vi "orientation_tester.vi"() -> ()   [LabVIEW 2026]
uses:
  <vilib>/Utility/error.llb/Trim Whitespace One-Sided.vi
panel:
  in  "Serial Port":refnum<visa-resource-name>="N/A"
  in  "stop":bool
  in  "Tab Control":enum32{"Integrated Circuit Testing"}(tab)
  out "Orientation OK":bool
  out "Detected IC":string
  out "Current":dbl(graph)
  in  "IC Select":u16(ring) items=["7408", "7432", "7404"]
  out "D1":bool
  out "D2":bool
  out "D3":bool
  out "D4":bool
  out "D5":bool
  out "D6":bool
  out "D8":bool
  out "D9":bool
  out "D10":bool
  out "D11":bool
  out "D12":bool
  out "D13":bool
  in  "Start Test":bool
  out "Tests Ran":dbl
  out "PASS":bool
  out "FAIL":bool
  out "Passed":dbl
  out "Failed":dbl
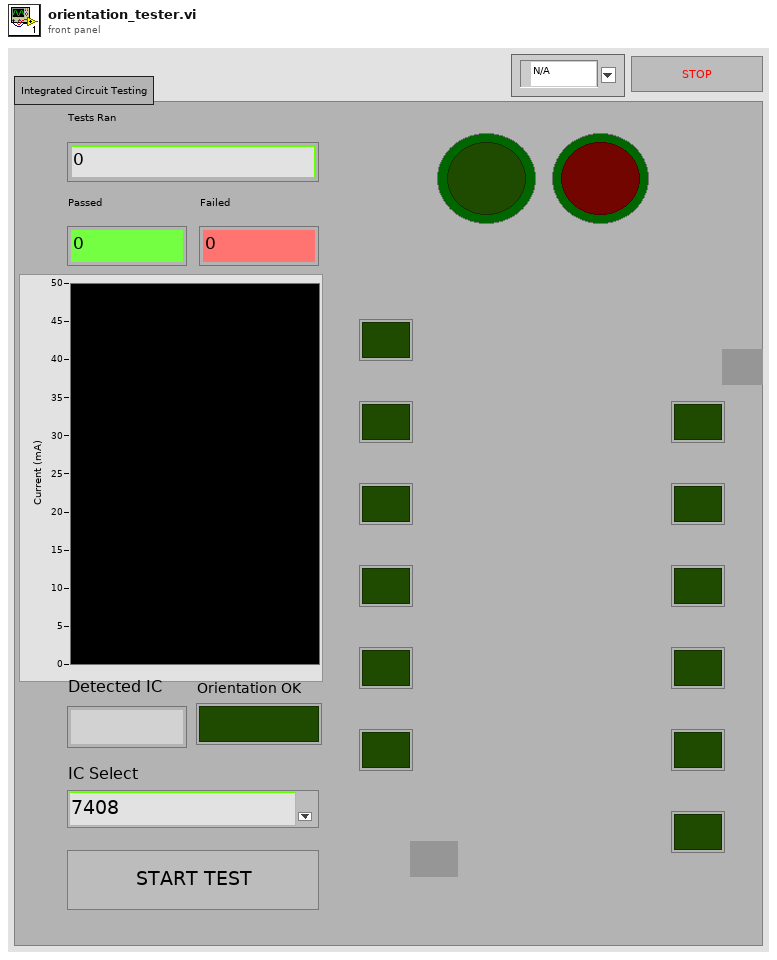
[diagram p1: front panel]
types:
  T1 = enum16{"Standard", "Buffered", "CRLF", "Immediate"}
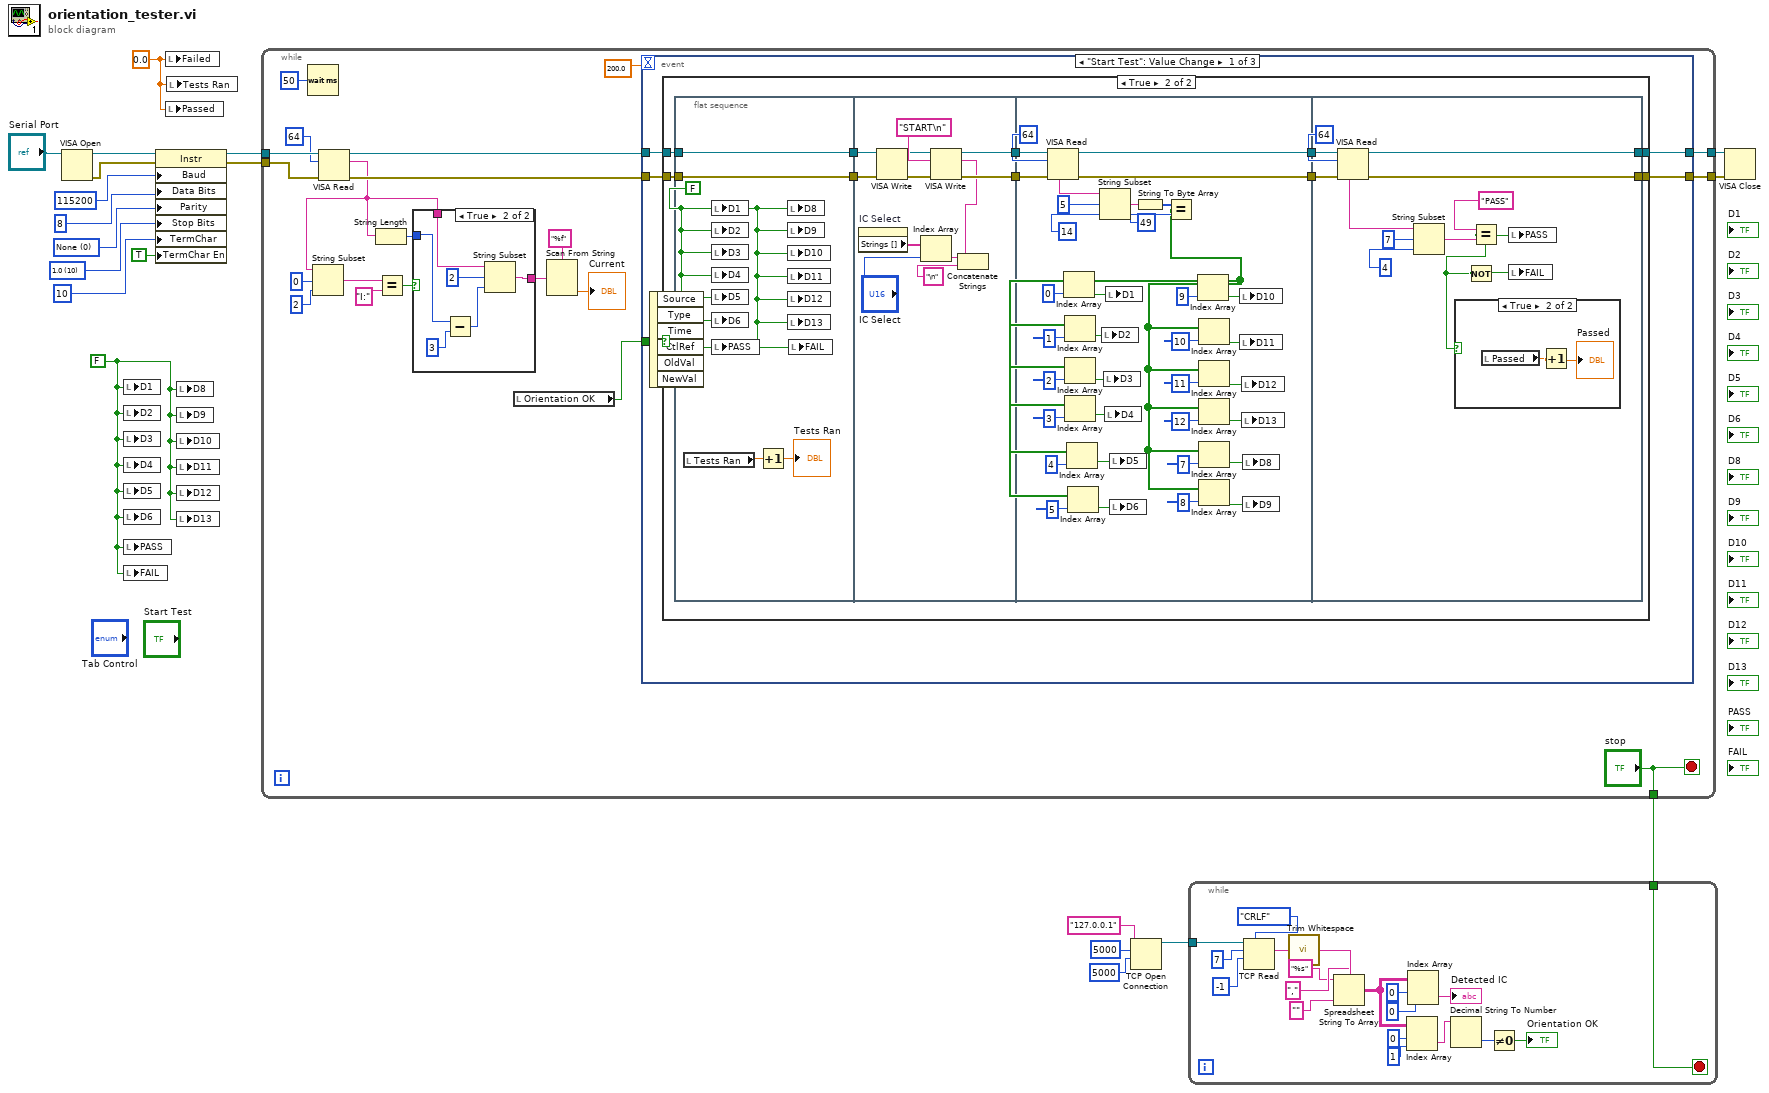
[diagram p0: block diagram]
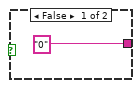
[diagram p2: hidden frame]
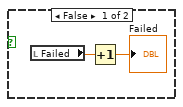
[diagram p4: hidden frame]
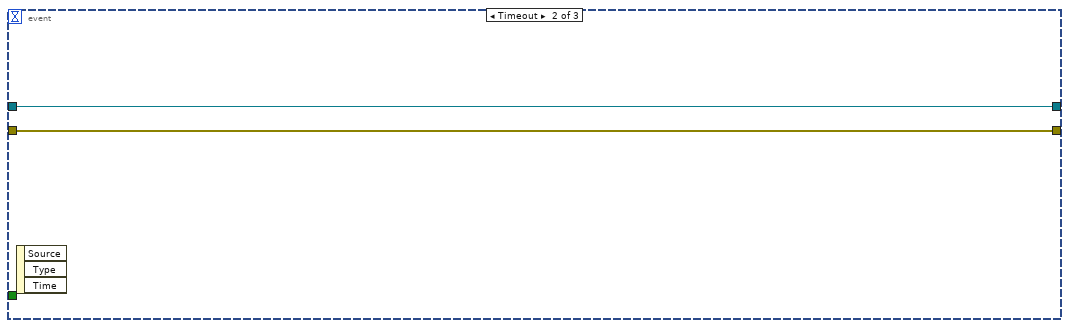
[diagram p5: hidden frame]
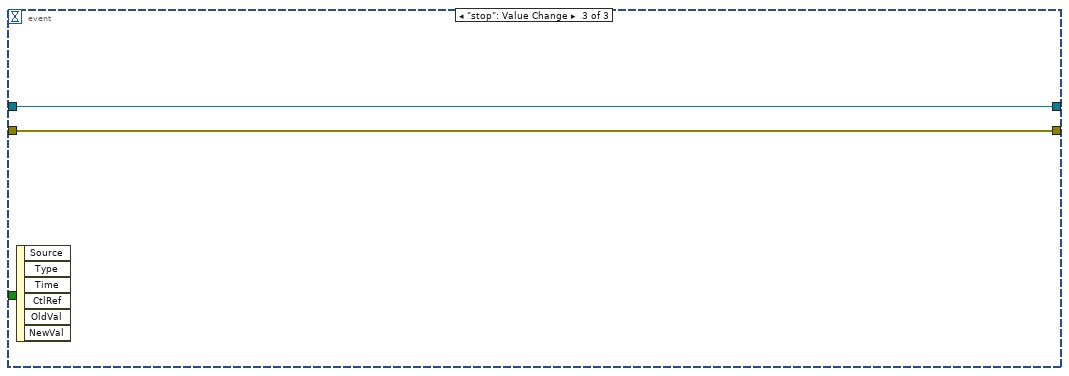
[diagram p6: hidden frame]
diagram:
  w3 = 0.0 ("Failed")
  w7 = FALSE ("D1")
  w12 = u16 10 items=["1.0"=10, "1.5"=15, "2.0"=20] ("Serial Settings:Stop Bits")
  w13 = u16 0 items=["None", "Odd", "Even", "Mark", "Space"] ("Serial Settings:Parity")
  n1 = VISA Open(VISA resource name="Serial Port") -> (VISA resource name=w19:refnum<visa-resource-name>, error out=w17:errorcluster)  [unwired: 4 in]
  n2 = local write "D1"(w7) -> ()
  n3 = local write "D2"(w7) -> ()
  n4 = local write "D3"(w7) -> ()
  n5 = local write "D4"(w7) -> ()
  n6 = local write "D5"(w7) -> ()
  n7 = local write "D6"(w7) -> ()
  n8 = local write "PASS"(w7) -> ()
  n9 = local write "FAIL"(w7) -> ()
  n10 = property class="Instr"(reference=w19, error in=w17, "Baud"=u32 115200 ("Serial Settings:Baud Rate"), "Data Bits"=u16 8 ("Serial Settings:Data Bits"), "Parity"=w13, "Stop Bits"=w12, "TermChar"=u8 10 ("Message Based Settings:Termination Character"), "TermChar En"=TRUE ("Message Based Settings:Termination Character Enable")) -> (reference out=w18:refnum<visa-resource-name>, error out=w16:errorcluster)
  n11 = local write "Failed"(w3) -> ()
  n12 = local write "Passed"(w3) -> ()
  n13 = local write "Tests Ran"(w3) -> ()
  n14 = local write "D8"(w7) -> ()
  n15 = local write "D9"(w7) -> ()
  n16 = local write "D10"(w7) -> ()
  n17 = local write "D11"(w7) -> ()
  n18 = local write "D12"(w7) -> ()
  n19 = local write "D13"(w7) -> ()
  n20 = while {
    tunnel: w18 -> [w41]
    tunnel: w16 -> [w39]
    tunnel: [w36] -> w9
    tunnel: [w35] -> w8
    tunnel: ["stop"] -> w1
    stop <- "stop" stop-if-true
    n21 = Wait (ms)(milliseconds to wait=u32 50) -> ()  [unwired: 1 out]
    n22 = VISA Read(VISA resource name=w41, byte count=u32 64, error in (no error)=w39) -> (VISA resource name out=w38:refnum<visa-resource-name>, read buffer=w29:string, error out=w37:errorcluster)  [unwired: 1 out]
    n23 = String Subset(string=w29, offset (0)=0, length (rest)=2 ("length (rest)")) -> (substring=w28:string)
    n24 = String Length(string=w29) -> (length=w30:i32)
    n25 = Equal?(x=w28, y="I:") -> (x = y?=w27:bool)
    n26 = case shown="True" w27 {
      tunnel: w30 -> [_ w47]
      tunnel: ["0" w44] -> w25
      tunnel: w29 -> [_ w43]
      frame False {
      }
      frame True {
        n27 = Subtract(x=w47, y=3) -> (x-y=w45:i32)
        n28 = String Subset(string=w43, offset (0)=2, length (rest)=w45) -> (substring=w44:string)
      }
    }
    n29 = local read "Orientation OK"() -> (w21:bool)
    n30 = Scan From String(format string="%f", input string=w25) -> (output 1=→"Current":dbl)  [unwired: 3 in, 3 out]
    n31 = event shown="[0] \"Start Test\": Value Change" {
      selector: _ -> [_ _ _]
      dyn-events: _ -> [_ _ _]
      timeout: 200.0 -> [_ _ _]
      tunnel: w38 -> [w53 w136 w138]
      tunnel: w37 -> [w52 w135 w137]
      tunnel: [w51 w136 w138] -> w36
      tunnel: [w50 w135 w137] -> w35
      tunnel: w21 -> [w49 _ _]
      event "Start Test": Value Change {
        n32 = event-data() -> ()  [unwired: 1 in, 6 out]
        n33 = case shown="True" w49 {
          tunnel: w53 -> [w55 w59]
          tunnel: w52 -> [w54 w58]
          tunnel: [w55 w57] -> w51
          tunnel: [w54 w56] -> w50
          frame False {
          }
          frame True {
            n34 = flat-sequence {
              tunnel: [w70] -> w65
              tunnel: w59 -> [w70]
              tunnel: [w69] -> w64
              tunnel: w58 -> [w69]
              tunnel: w65 -> [w79]
              tunnel: w64 -> [w77]
              tunnel: [w82] -> w63
              tunnel: [w81] -> w62
              tunnel: w63 -> [w117]
              tunnel: w62 -> [w118]
              tunnel: [w116] -> w61
              tunnel: [w115] -> w60
              tunnel: [w127] -> w56
              tunnel: [w128] -> w57
              tunnel: w61 -> [w130]
              tunnel: w60 -> [w129]
              frame #0 {
                w68 = FALSE ("D1")
                n35 = local read "Tests Ran"() -> (w67:dbl)
                n36 = local write "D1"(w68) -> ()
                n37 = local write "D2"(w68) -> ()
                n38 = local write "D3"(w68) -> ()
                n39 = local write "D4"(w68) -> ()
                n40 = local write "D5"(w68) -> ()
                n41 = local write "D6"(w68) -> ()
                n42 = local write "PASS"(w68) -> ()
                n43 = Increment(x=w67) -> (x+1=→"Tests Ran":dbl)
                n44 = local write "D8"(w68) -> ()
                n45 = local write "D9"(w68) -> ()
                n46 = local write "D10"(w68) -> ()
                n47 = local write "D11"(w68) -> ()
                n48 = local write "D12"(w68) -> ()
                n49 = local write "D13"(w68) -> ()
                n50 = local write "FAIL"(w68) -> ()
              }
              frame #1 {
                n51 = property on="IC Select" class="Ring (strict)"() -> ("Strings []"=w75:string[])  [unwired: 2 in, 2 out]
                n52 = Index Array(array=w75, index="IC Select") -> (element=w73:string)
                n53 = Concatenate Strings(w73, "\n" ("string")) -> (w71:string)
                n54 = VISA Write(VISA resource name=w79, write buffer=w71, error in (no error)=w77) -> (VISA resource name out=w78:refnum<visa-resource-name>, error out=w76:errorcluster)  [unwired: 1 out]
                n55 = VISA Write(VISA resource name=w78, write buffer="START\n", error in (no error)=w76) -> (VISA resource name out=w82:refnum<visa-resource-name>, error out=w81:errorcluster)  [unwired: 1 out]
              }
              frame #2 {
                n56 = VISA Read(VISA resource name=w117, byte count=u32 64, error in (no error)=w118) -> (VISA resource name out=w116:refnum<visa-resource-name>, read buffer=w109:string, error out=w115:errorcluster)  [unwired: 1 out]
                n57 = String Subset(string=w109, offset (0)=5, length (rest)=14 ("length (rest)")) -> (substring=w113:string)
                n58 = String To Byte Array(string=w113) -> (unsigned byte array=w112:u8[])
                n59 = Equal?(x=w112, y=u8 49) -> (x = y?=w84:bool[])
                n60 = Index Array(array=w84, index=0) -> (element=w108:bool)
                n61 = Index Array(array=w84, index=1) -> (element=w104:bool)
                n62 = Index Array(array=w84, index=2) -> (element=w103:bool)
                n63 = Index Array(array=w84, index=3) -> (element=w106:bool)
                n64 = Index Array(array=w84, index=4) -> (element=w107:bool)
                n65 = Index Array(array=w84, index=5) -> (element=w105:bool)
                n66 = local write "D2"(w104) -> ()
                n67 = local write "D3"(w103) -> ()
                n68 = local write "D4"(w106) -> ()
                n69 = local write "D1"(w108) -> ()
                n70 = local write "D5"(w107) -> ()
                n71 = local write "D6"(w105) -> ()
                n72 = Index Array(array=w84, index=9) -> (element=w94:bool)
                n73 = Index Array(array=w84, index=10) -> (element=w93:bool)
                n74 = Index Array(array=w84, index=11) -> (element=w92:bool)
                n75 = Index Array(array=w84, index=12) -> (element=w91:bool)
                n76 = Index Array(array=w84, index=7) -> (element=w96:bool)
                n77 = Index Array(array=w84, index=8) -> (element=w95:bool)
                n78 = local write "D10"(w94) -> ()
                n79 = local write "D11"(w93) -> ()
                n80 = local write "D12"(w92) -> ()
                n81 = local write "D13"(w91) -> ()
                n82 = local write "D8"(w96) -> ()
                n83 = local write "D9"(w95) -> ()
              }
              frame #3 {
                n84 = VISA Read(VISA resource name=w130, byte count=u32 64, error in (no error)=w129) -> (VISA resource name out=w128:refnum<visa-resource-name>, read buffer=w123:string, error out=w127:errorcluster)  [unwired: 1 out]
                n85 = String Subset(string=w123, offset (0)=7, length (rest)=4 ("length (rest)")) -> (substring=w119:string)
                n86 = Equal?(x="PASS", y=w119) -> (x = y?=w120:bool)
                n87 = case shown="True" w120 {
                  frame False {
                    n88 = local read "Failed"() -> (w131:dbl)
                    n89 = Increment(x=w131) -> (x+1=→"Failed":dbl)
                  }
                  frame True {
                    n90 = local read "Passed"() -> (w133:dbl)
                    n91 = Increment(x=w133) -> (x+1=→"Passed":dbl)
                  }
                }
                n92 = Not(x=w120) -> (.not. x?=w122:bool)
                n93 = local write "PASS"(w120) -> ()
                n94 = local write "FAIL"(w122) -> ()
              }
            }
          }
        }
      }
      event Timeout {
        n95 = event-data() -> ()  [unwired: 1 in, 3 out]
      }
      event "stop": Value Change {
        n96 = event-data() -> ()  [unwired: 1 in, 6 out]
      }
    }
  }
  n97 = TCP Open Connection(address="127.0.0.1", remote port or service name=u16 5000, timeout ms (60000)=5000) -> (connection ID=w2:refnum<k5>)  [unwired: 2 in, 1 out]
  n98 = while {
    tunnel: w2 -> [w140]
    tunnel: w1 -> [w139]
    stop <- w139 stop-if-true
    n99 = TCP Read(connection ID=w140, bytes to read=7, 7:T1."CRLF" ("mode (standard)"), 9:-1 ("timeout ms (25000)")) -> (data out=w152:string)  [unwired: 1 in, 2 out]
    n100 = call <vilib>:"Trim Whitespace.vi"("string"=w152) -> ("trimmed string"=w153:string)  [unwired: 1 in]
    n101 = Spreadsheet String To Array(delimiter (Tab)=",", format string="%s", spreadsheet string=w153, array type (2D Dbl)="") -> (array=w154:string[][])
    n102 = Index Array(array=w154, index (row)=0, index (col)=1 ("disabled index (col)")) -> (element=w157:string)
    n103 = Index Array(array=w154, index (row)=0, index (col)=0 ("disabled index (col)")) -> (element=→"Detected IC":string)
    n104 = Decimal String To Number(string=w157) -> (number=w156:i32)  [unwired: 2 in, 1 out]
    n105 = Not Equal To 0?(x=w156) -> (x != 0?=→"Orientation OK":bool)
  }
  n106 = VISA Close(VISA resource name=w9, error in (no error)=w8) -> ()  [unwired: 1 out]
